vi "CLIENT_initialize_manual_editors.vi"(8 "error_in":errorcluster, 11 "all_config_info":T1={"main_ini_file"={"SQL Driver"="", "SQL Server"="", "SQL Database"="", "SQL UID"="", "Reference table"="", "Reference history"="", "Archivisation CFG table"="", "Archivisation CFG history"="", "User table"="", "User history"="", "logout timeout [ms]"=0, "records per page"=0, "default language"="", "REF CHG connection IP"="", "REF CHG remote port"=0, "REF CHG local port"=0, "SCANNER COM port"=0, "SCANNER Baud rate"=0, "SCANNER Data bits"=0, "SCANNER Pairity"=enum."None", "SCANNER Stop bits"=10, "SCANNER Flow control"=0, "SCANNER Termination char"=0}, "SQL Password"="", "queue_refnums"={"SQL_EDITOR_queue"=refnum, "SCANNER_queue"=refnum, "SCANNER_data"=refnum, "CLIENT_REF_CHG_queue"=refnum}} {"main_ini_file"."SCANNER Flow control" items=["None"=0, "XON/XOFF"=1, "RTS/CTS"=2, "DTR/DSR"=4]; "main_ini_file"."SCANNER Stop bits" items=["1.0"=10, "1.5"=15, "2.0"=20]}) -> (0 "error_out":errorcluster)   [LabVIEW 2019]
uses:
  ini/typedef/CLIENT_all_config_info.ctl
  ini/typedef/CLIENT_main_ini_file.ctl
  queues/typedef/CLIENT_queue_refnums.ctl
  queues/typedef/SQL_EDITOR_queue_element.ctl
  MAIN/SQL_EDITOR/SQL_EDITOR_sequence_state.ctl
  queues/typedef/CLIENT_SCANNER_queue_element.ctl
  MAIN/SCANNER/SCANNER_sequence_state.ctl
  queues/typedef/CLIENT_REF_CHG_queue_element.ctl
  MAIN/reference_changed_connection/CLIENT_REF_CHG_sequence_state.ctl
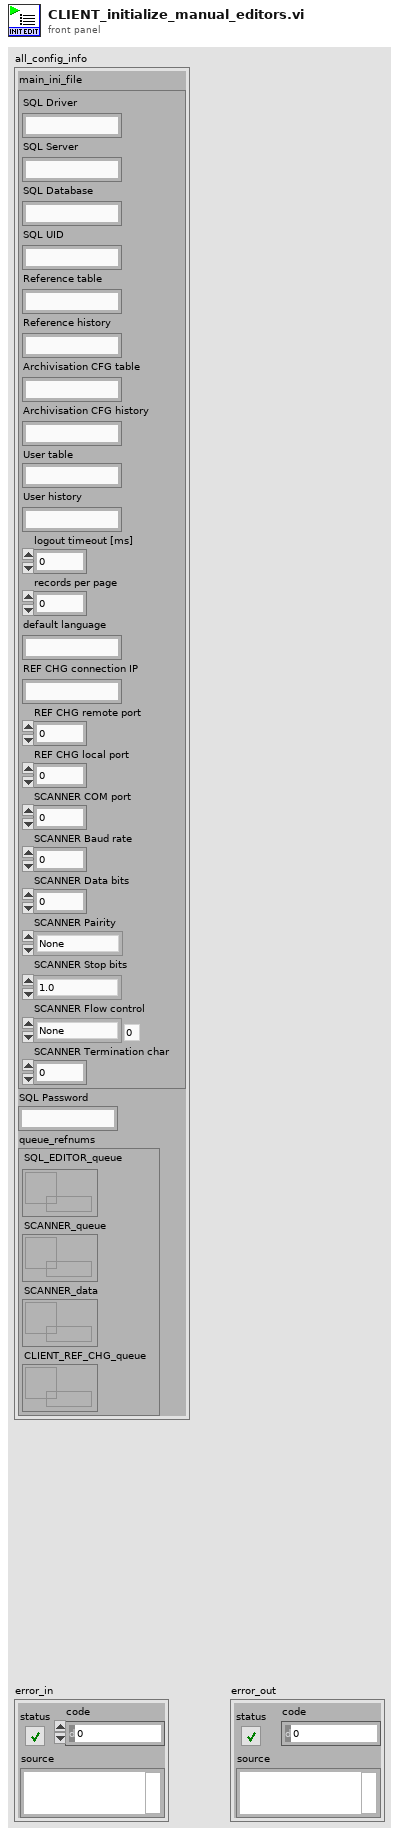
[diagram p1: front panel]
types:
  T1 = typedef "CLIENT_all_config_info.ctl" = cluster{"main_ini_file":T2, "SQL Password":string, "queue_refnums":T3}
  T2 = typedef "CLIENT_main_ini_file.ctl" = cluster{"SQL Driver":string, "SQL Server":string, "SQL Database":string, "SQL UID":string, "Reference table":string, "Reference history":string, "Archivisation CFG table":string, "Archivisation CFG history":string, "User table":string, "User history":string, "logout timeout [ms]":i32, "records per page":i32, "default language":string, "REF CHG connection IP":string, "REF CHG remote port":i32, "REF CHG local port":i32, "SCANNER COM port":u16, "SCANNER Baud rate":u32, "SCANNER Data bits":u16, "SCANNER Pairity":enum16{"None", "Odd", "Even", "Mark", "Space"}, "SCANNER Stop bits":u16, "SCANNER Flow control":u16, "SCANNER Termination char":u8}
  T3 = typedef "CLIENT_queue_refnums.ctl" = cluster{"SQL_EDITOR_queue":refnum<queue>, "SCANNER_queue":refnum<queue>, "SCANNER_data":refnum<queue>, "CLIENT_REF_CHG_queue":refnum<queue>}
  T4 = typedef "SQL_EDITOR_queue_element.ctl" = cluster{"state":T5, "variable":variant}
  T5 = typedef "SQL_EDITOR_sequence_state.ctl" = enum16{"initialize", "get_next_state", "REF_read_columns", "REF_read_stations", "REF_select_station_records", "REF_insert_record", "REF_update_record", "REF_delete_record", "REF_send_reference_updated_to_PLC", "ARCH_read_columns", "ARCH_read_stations", "ARCH_select_station_records", "ARCH_insert_record", "ARCH_update_record", "ARCH_delete_record", "USER_read_columns", "USER_select_records", "USER_insert_record", "USER_update_record", "USER_delete_record", "USER_update_barcode", "USER_login", "USER_logout", "SQL_read_tables", "SQL_read_columns", "SQL_select_records", "SQL_insert_record", "SQL_update_record", "SQL_delete_record", "SQL_TEXT_execute", "REPORT_GEAR_scan_barcode", "REPORT_GEAR_get", "REPORT_DATES_get", "REPORT_PBATCH_get", "REPORT_OPRTN_get", "REPORT_CFG_get", "REPORT_AUDIT_get", "REPORT_OKNOK_get", "REPORT_REWORKS_get", "REPORT_PACE_get", "REPORT_CBATCH_scan_barcode", "REPORT_CBATCH_get", "REPORT_CMPNT_scan_barcode", "REPORT_CMPNT_get", "REPORT_save_pdf", "REPORT_save_csv", "error", "stop"}
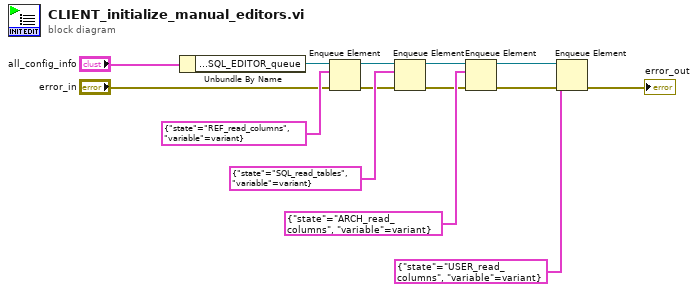
[diagram p0: block diagram]
diagram:
  n1 = Unbundle By Name("all_config_info") -> ("queue_refnums.SQL_EDITOR_queue"=w9:refnum<queue>)
  n2 = Enqueue Element(queue=w9, element=T4 {"state"=enum."REF_read_columns", "variable"=variant}, error in (no error)="error_in") -> (queue out=w10:refnum<queue>, error out=w6:errorcluster)  [unwired: 1 in, 1 out]
  n3 = Enqueue Element(queue=w10, element=T4 {"state"=enum."SQL_read_tables", "variable"=variant}, error in (no error)=w6) -> (queue out=w13:refnum<queue>, error out=w7:errorcluster)  [unwired: 1 in, 1 out]
  n4 = Enqueue Element(queue=w13, element=T4 {"state"=enum."ARCH_read_columns", "variable"=variant}, error in (no error)=w7) -> (queue out=w2:refnum<queue>, error out=w4:errorcluster)  [unwired: 1 in, 1 out]
  n5 = Enqueue Element(queue=w2, element=T4 {"state"=enum."USER_read_columns", "variable"=variant}, error in (no error)=w4) -> (error out=→"error_out":errorcluster)  [unwired: 1 in, 2 out]
